vi "predict_logic.vi"(7 "thres_signal":dbl, 8 "release":bool, 9 "time_offset(msec)":dbl, 10 "input_signal":dbl) -> (1 "control_enable":bool, 2 "predict signal":dbl)   [LabVIEW 2020]
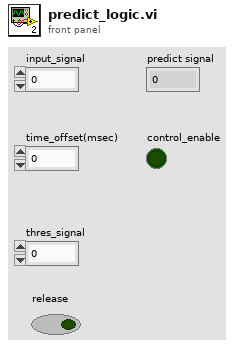
[diagram p1: front panel]
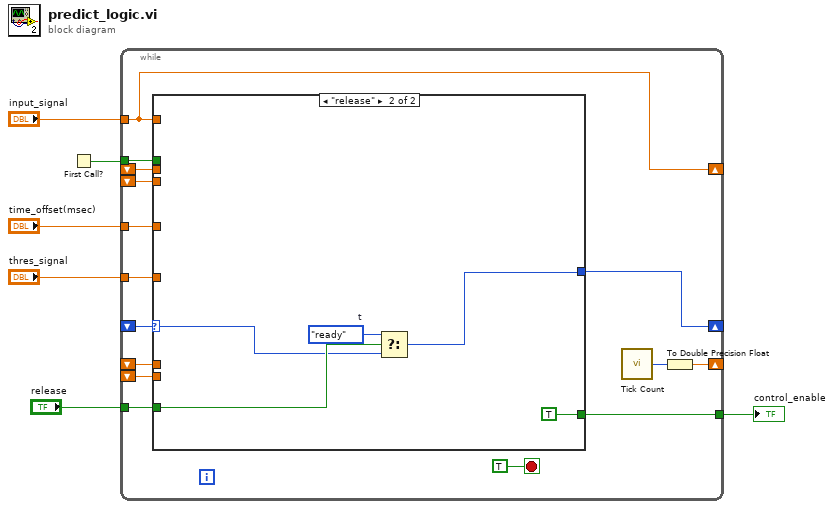
[diagram p0: block diagram]
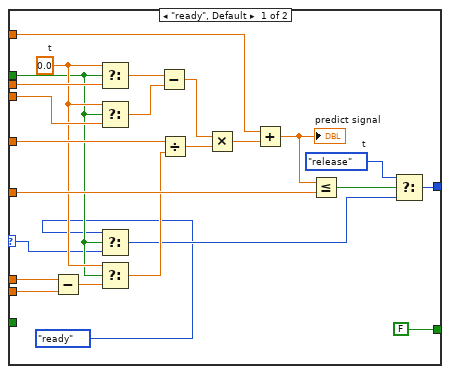
[diagram p2: hidden frame]
diagram:
  n1 = First Call?() -> (First Call?: T/F=w3:bool)
  n2 = while {
    shift-right: [w9] -> _
    shift-left: _ -> [w20]
    shift-left: _ -> [w19]
    tunnel: "time_offset(msec)" -> [w15]
    tunnel: "input_signal" -> [w9]
    tunnel: "thres_signal" -> [w18]
    tunnel: w3 -> [w14]
    shift-right: [w10] -> _
    shift-left: _ -> [w17]
    shift-left: _ -> [w16]
    shift-right: [w12] -> _
    shift-left: _ -> [w13]
    tunnel: [w8] -> w2
    tunnel: "release" -> [w7]
    stop <- TRUE stop-if-true
    n3 = case shown="\"release\"" w13 {
      selector: w13 -> [w24 w48]
      tunnel: w20 -> [w43 _]
      tunnel: w19 -> [w42 _]
      tunnel: w9 -> [w31 _]
      tunnel: w18 -> [w38 _]
      tunnel: w17 -> [w37 _]
      tunnel: w16 -> [w36 _]
      tunnel: w15 -> [w34 _]
      tunnel: w14 -> [w25 _]
      tunnel: [w28 w47] -> w12
      tunnel: [FALSE TRUE] -> w8
      tunnel: w7 -> [_ w49]
      frame "ready", Default {
        w29 = enum16{"ready", "release"}."release"  # t
        w32 = 0.0  # t
        n4 = Subtract(x=w37, y=w36) -> (x-y=w35:dbl)
        n5 = Select(t=w32, s=w25, f=w43) -> (s? t:f=w41:dbl)
        n6 = Select(t=w32, s=w25, f=w42) -> (s? t:f=w40:dbl)
        n7 = Select(t=enum16{"ready", "release"}."ready", s=w25, f=w24) -> (s? t:f=w23:enum16{"ready", "release"})
        n8 = Select(t=w32, s=w25, f=w35) -> (s? t:f=w26:dbl)
        n9 = Subtract(x=w41, y=w40) -> (x-y=w39:dbl)
        n10 = Divide(x=w34, y=w26) -> (x/y=w33:dbl)
        n11 = Multiply(x=w39, y=w33) -> (x*y=w45:dbl)
        n12 = Add(x=w31, y=w45) -> (x+y=w44:dbl)
        "predict signal" <- w44
        n13 = Less Or Equal?(x=w44, y=w38) -> (x <= y?=w30:bool)
        n14 = Select(t=w29, s=w30, f=w23) -> (s? t:f=w28:enum16{"ready", "release"})
      }
      frame "release" {
        w46 = enum16{"ready", "release"}."ready"  # t
        n15 = Select(t=w46, s=w49, f=w48) -> (s? t:f=w47:enum16{"ready", "release"})
      }
    }
    n16 = call "Tick Count"() -> ("Tick Count(mSec)"=w11:u32)
    n17 = To Double Precision Float(number=w11) -> (double precision float=w10:dbl)
  }
  "control_enable" <- w2
